vi "ReadDataFile.vi"(10 "File Paths":T1={"Local Save Path"=path "\\\\smbhome.uscs.susx.ac.uk\\cv222/Desktop/data", "Newton Save Path"=path "Z:/#Projects/Entanglement/data", "File Name"="test", "LocalSave"=TRUE}) -> (0 "params":string, 1 "runs":i32, 2 "All data":dbl[][](array[numeric]), 3 "Last run data":dbl[][](array[numeric]))   [LabVIEW 2017]
uses:
  controls/FilePaths.ctl
  controls/GlobalExp.vi
  <vilib>/Utility/file.llb/Read From Spreadsheet File (string).vi
  Global.lvlib
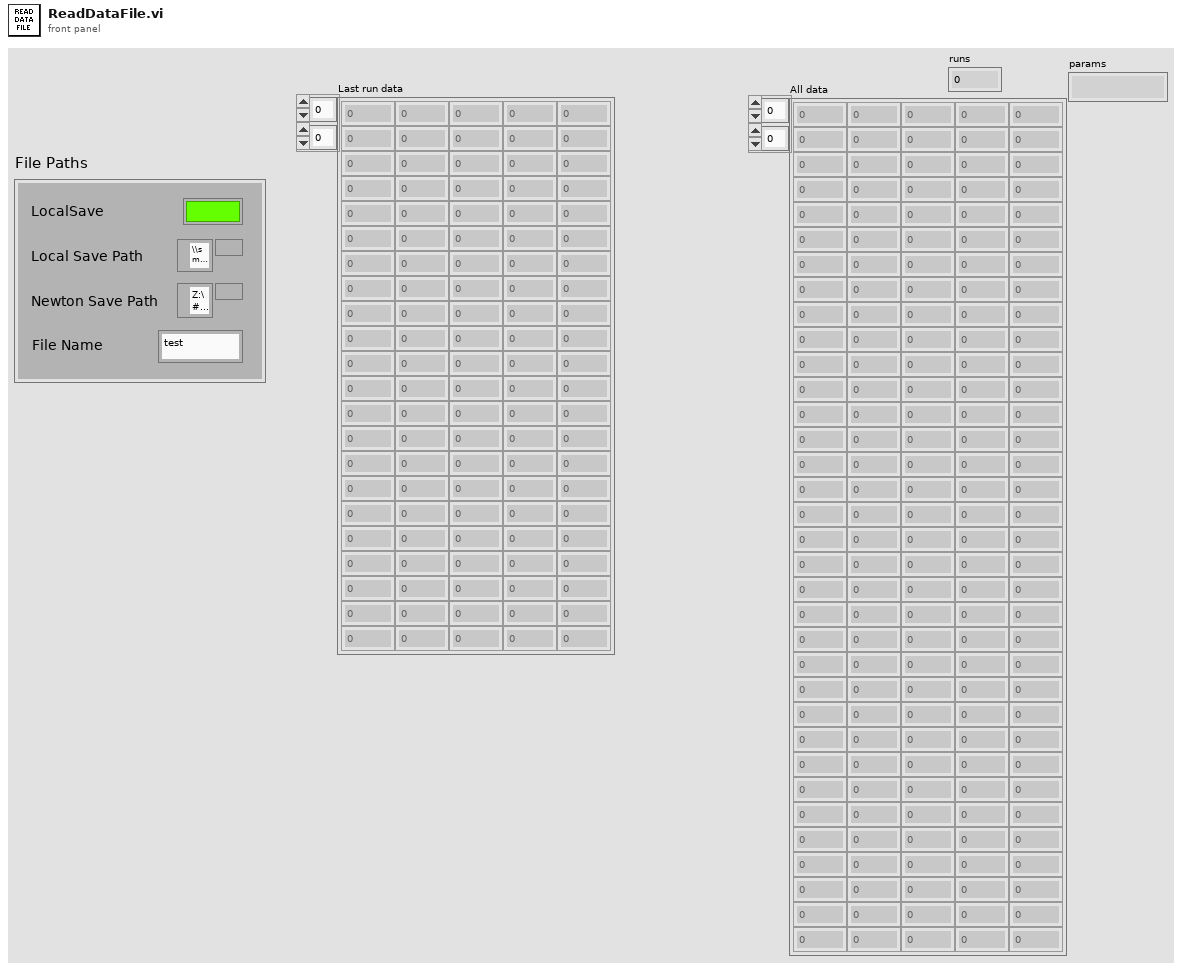
[diagram p1: front panel]
types:
  T1 = typedef "FilePaths.ctl" = cluster{"Local Save Path":path, "Newton Save Path":path, "File Name":string, "LocalSave":bool}
  T2 = typedef "MasterExpControl.ctl" = cluster{"Main Steps":dbl, "Main Runs":dbl, "ExpStatus":enum16{"Innit", "Stop", "Idle", "MainRunning", "AuxRunning"}, "Main Current Step":dbl, "ExpNum":dbl, "NewData":bool, "date":string, "command":string, "Stop":bool, "Pause":bool, "Mathematica":string, "Main/Meta":bool, "UpdateMath":bool, "Camera":bool}
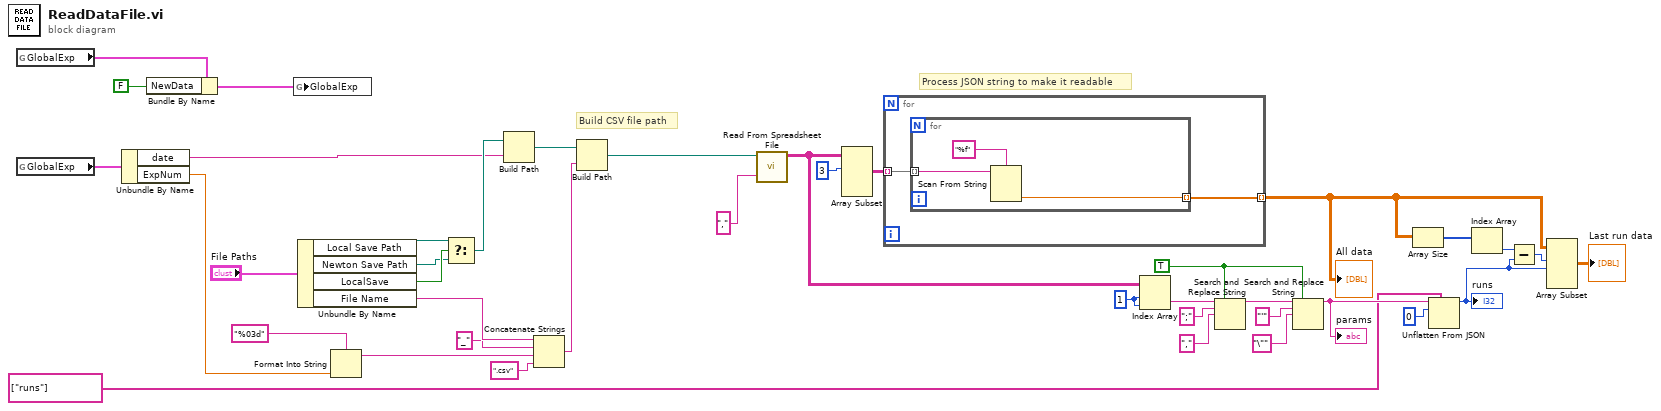
[diagram p0: block diagram]
diagram:
  w31 = TRUE ("replace all? (F)")
  w22 = 1 ("index (row)")
  # "Process JSON string to make it readable"
  # "Build CSV file path"
  n1 = global read "GlobalExp.vi" "GlobalExp"() -> (w16:T2)
  n2 = global read "GlobalExp.vi" "GlobalExp"() -> (w8:T2)
  n3 = Unbundle By Name(w8) -> ("date"=w6:string, "ExpNum"=w9:dbl)
  n4 = Bundle By Name(cluster=w16, "NewData"=FALSE) -> (w10:T2)
  n5 = global write "GlobalExp.vi" "GlobalExp"(w10) -> ()
  n6 = Unbundle By Name("File Paths") -> ("Local Save Path"=w36:path, "Newton Save Path"=w37:path, "LocalSave"=w38:bool, "File Name"=w40:string)
  n7 = Format Into String(format string="%03d", w9) -> (resulting string=w2:string)  [unwired: 2 in, 1 out]
  n8 = Select(t=w36, s=w38, f=w37) -> (s? t:f=w39:path)
  n9 = Build Path(base path=w39, name or relative path=w6) -> (appended path=w7:path)
  n10 = Concatenate Strings(w40, "_", w2, ".csv") -> (w4:string)
  n11 = Build Path(base path=w7, name or relative path=w4) -> (appended path=w12:path)
  n12 = call-poly <vilib>:"Read From Spreadsheet File.vi"("delimiter (\\t)"="," ("delimiter (\\t)"), "file path (dialog if empty)"=w12) -> ("all rows"=w21:string[][])  [unwired: 5 in, 4 out]
  n13 = Array Subset(array=w21, index (row)=3 ("index")) -> (w15:string[][])  [unwired: 3 in]
  n14 = for {
    tunnel: w15 -> [w42] mode=indexing
    tunnel: [w41] -> w17 mode=indexing
    n15 = for {
      tunnel: w42 -> [w45] mode=indexing
      tunnel: [w43] -> w41 mode=indexing
      n16 = Scan From String(format string="%f", input string=w45) -> (output 1=w43:dbl)  [unwired: 3 in, 3 out]
    }
  }
  "All data" <- w17
  n17 = Index Array(array=w21, index (row)=w22, index (col)=w22) -> (element=w32:string)
  n18 = Search and Replace String(replace all?=w31, input string=w32, search string=";", replace string="," ("replace string (\"\")")) -> (result string=w28:string)  [unwired: 4 in, 3 out]
  n19 = Search and Replace String(replace all?=w31, input string=w28, search string="'", replace string="\"" ("replace string (\"\")")) -> (result string=w33:string)  [unwired: 4 in, 3 out]
  "params" <- w33
  n20 = Array Size(array=w17) -> (size(s)=w18:i32[])
  n21 = Unflatten From JSON(path=string[] ["runs"], JSON string=w33, type and defaults=0) -> (value=w25:i32)  [unwired: 4 in, 1 out]
  "runs" <- w25
  n22 = Index Array(array=w18) -> (element=w19:i32)  [unwired: 1 in]
  n23 = Subtract(x=w19, y=w25) -> (x-y=w20:i32)
  n24 = Array Subset(array=w17, index (row)=w20, length (row)=w25) -> (→"Last run data":dbl[][])  [unwired: 2 in]
